vi "Try Parse.vi"(0 "Vector Path in":refnum<class "Vector Path.lvclass">, 5 "Config Row":string[](array[string]), 11 "error in (no error)":errorcluster) -> (4 "Vector Path out":refnum<class "Vector Path.lvclass">, 6 "Is of type?":bool, 15 "error out":errorcluster)   [LabVIEW 2023, in "RFFixtureCharact.Public.lvlib" / "Vector Path.lvclass"]
uses:
  Vector Path.lvclass
  Vector Path.lvclass/Vector Path.ctl
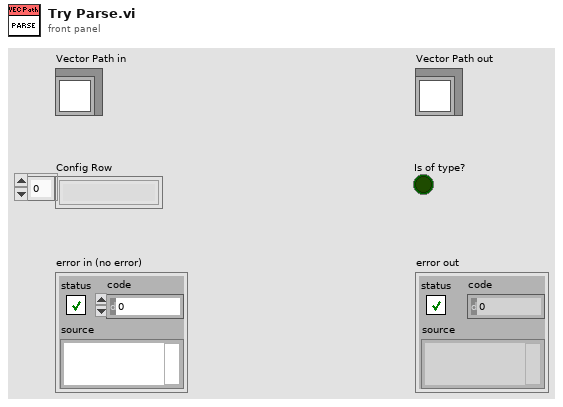
[diagram p1: front panel]
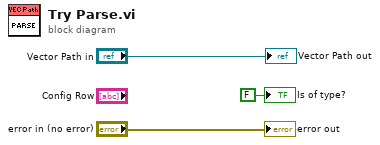
[diagram p0: block diagram]
diagram:
  "error out" <- "error in (no error)"
  "Vector Path out" <- "Vector Path in"
  "Is of type?" <- FALSE ("Is of type?")
